vi "Write to File.vi"(8 "error in (no error)":errorcluster, 11 "TDMS Report in":refnum<class "TDMS Report - Solution.lvclass">) -> (0 "error out":errorcluster, 3 "TDMS Report out":refnum<class "TDMS Report - Solution.lvclass">)   [LabVIEW 2011, in "TDMS Report - Solution.lvclass"]
doc: "Part of the solution for the TDMS Report Object. This is a dynamic dispatch VI that overrides the associated method in the parent.\n\nAAL 9/09"
uses:
  TDMS Report - Solution.lvclass
  Report Class/Report.lvclass
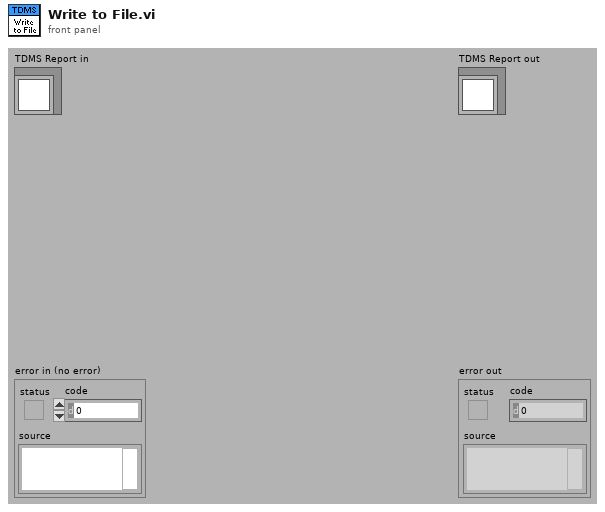
[diagram p1: front panel]
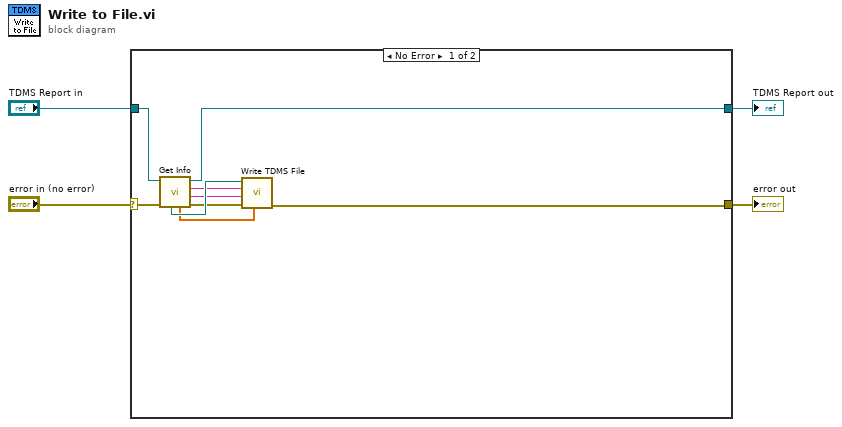
[diagram p0: block diagram]
diagram:
  n1 = case shown="No Error" "error in (no error)" {
    selector: "error in (no error)" -> [w11 w15]
    tunnel: [w8 w15] -> w3
    tunnel: [w12 w14] -> w1
    tunnel: "TDMS Report in" -> [w13 w14]
    frame No Error {
      n2 = call "Get Info.vi"("error in (no error)"=w11, "Report"=w13) -> ("error out"=w9:errorcluster, "Data & Time String"=w6:string, "Header"=w7:string, "Report out"=w12:refnum<class "TDMS Report - Solution.lvclass">, "Data Array"=w5:dbl[], "Path"=w10:path)  [unwired: 4 out]
      n3 = call "Write TDMS File.vi"("Data Array"=w5, "error in"=w9, "Data & Time String"=w6, "Header"=w7, "Path"=w10) -> ("error out"=w8:errorcluster)  [unwired: 6 in]
    }
    frame Error {
    }
  }
  "error out" <- w3
  "TDMS Report out" <- w1
